vi "Polynomial Roots.vi"   [LabVIEW 2024, in "NI_AALPro.lvlib"]
doc: "<p>Finds the roots of polynomial <strong>P(x)</strong>. This VI removes leading coefficients of the polynomial that are equal to zero. Wire data to the <strong>P(x)</strong> input to determine the polymorphic instance to use or <a href=\"nihelplauncher://docs/csh?context=lvcore_lvhowto_selectingdefaultinstpolyvi\">manually select</a> the instance.</p>"
uses:
  NI_AALPro.lvlib
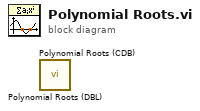
[diagram p0: block diagram]
diagram:
  n1 = call "Polynomial Roots (DBL).vi"() -> ()  [unwired: 10 in, 2 out]
  n2 = call "Polynomial Roots (CDB).vi"() -> ()  [unwired: 10 in, 2 out]
